vi "PTSequencer.add step.vi"(0 "i ref in":refnum<vi>, 2 "Step":T1, 3 "ms timeout (10000)":i32=10000, 5 "error in (no error)":errorcluster) -> (14 "i ref out":refnum<vi>, 17 "timed out":bool, 19 "error out":errorcluster)   [LabVIEW 2014, in "PTSequencer.lvlib"]
uses:
  PTSequencer.lvlib
  PTSequencer.step.ctl
  CS_Core/CSSystem/CoreDefs/CoreDefs.rawDataType.ctl
  PTSequencer.DIM service condition.ctl
  CS_Core/CSSystem/CoreDefs/CoreDefs.error_type.ctl
  CS_Core/CSSystem/CoreDefs/CoreDefs.error_severity.ctl
  CS_Core/CSSystem/CSSystemLib/CSSystemLib.lvlib
  CS_Core/CSSystem/CoreLib/CoreLib.lvlib
  CS_Core/CSSystem/CoreLib/CoreLib.string 2 byte array.vi
  CS_Core/BaseProcess/BaseProcess.lvlib
  CS_Core/CSSystem/CoreLib/CoreLib.byte array 2 short.vi
  CSlibraries/UtilityLib/UtilityLib.lvlib
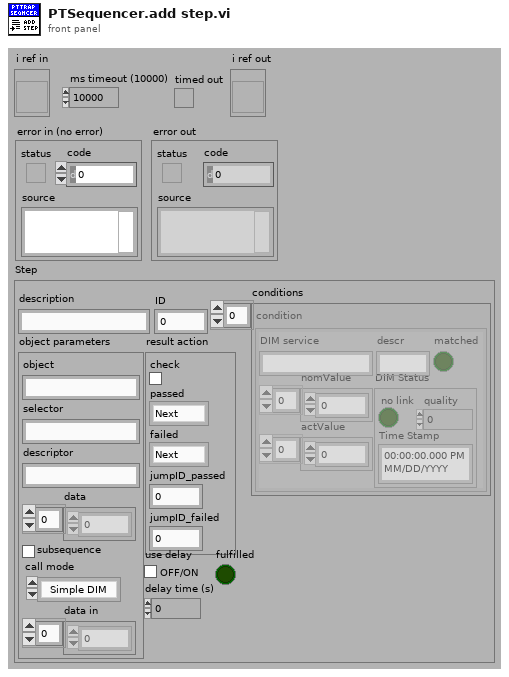
[diagram p1: front panel]
types:
  T1 = typedef "PTSequencer.lvlib/PTSequencer.step.ctl" = cluster{"description":string, "object parameters":cluster{"object":string, "selector":string, "descriptor":string, "data":T2, "subsequence":bool, "call mode":enum16{"Simple DIM", "Synchronous"}, "data in":T2}, "result action":cluster{"check":bool, "passed":enum16{"Next", "Previous", "Repeat", "Jump"}, "failed":enum16{"Next", "Previous", "Repeat", "Jump"}, "jumpID_passed":i32, "jumpID_failed":i32}, "conditions":T3[], "fulfilled ":bool, "use delay":bool, "delay time (s)":dbl, "ID":i32}
  T2 = typedef "CoreDefs.rawDataType.ctl" = i8[]
  T3 = typedef "PTSequencer.lvlib/PTSequencer.DIM service condition.ctl" = cluster{"DIM service":string, "descr":string, "nomValue":T2, "actValue":T2, "matched":bool, "DIM Status":cluster{"no link":bool, "quality":i32, "Time Stamp":timestamp}}
  T4 = typedef "CoreDefs.error_severity.ctl" = enum16{"undefined", "information", "warning", "error", "fatal"}
  T5 = typedef "CoreDefs.error_type.ctl" = enum16{"no error", "can't load process", "can't unload process", "process does not exist", "can't install process", "can't remove process", "unknown function", "time out", "can't execute function", "duplicate queue name", "super not found", "caller queue invalid", "can't ping process", "unknown error", "VISA Error", "VISA timeout", "GPIB timeout", "GPIB error", "communication error", "data type mismatch", "can't read data from OPC server", "can't write data to OPC server", "OET error", "function not implemented", "process already exists", "invalid Shared Variable name", "error writing Shared Variable", "error reading Shared Variable", "invalid client name", "corrupt database", "unknown class", "call not authorized", "parameter out of range", "OET timeout: can't get data to modify", "invalid queue name", "requested operation incompatible with current state", "event undefined", "event disabled", "state undefined", "caller is not a friend", "EventBuilder: bad eventID", "EventBuilder: no DAQ devices", "a thread must not stop itself", "UNUSED ELEMENT4", "DiscArchiver: eventData incomplete", "DiscArchiver: eventData does not belong to run", "DiscArchiver: can't open file", "DiscArchiver: can't write to file", "DiscArchiver: available disc space low", "can't acquire semaphore", "error reading data from database", "notifier object is not existing", "can't register process", "can't unregister process", "illegal event type", "object disabled", "object already exists", "can't change state", "Instrument not found", "no connection to remote node", "invalid reference", "N/A", "UNUSED ELEMENT 1", "element not found", "illegal TCP/IP connection detected", "object does not exist", "invalid access ID", "unknown CS system", "invalid privilige", "unsupported data type", "unsupported server type", "IO server already exists", "Shared Variable already exists"}
  T6 = typedef "PTSequencer.lvlib/PTSequencer.i attribute.ctl" = cluster{"subsequence":bool, "mode":T7, "i step":i32, "nofLoops":i32, "i loop":i32, "Running":bool, "Paused":bool, "step done":bool, "loop done":bool, "seq done":bool, "DIM IDs":cluster{"step done":i32, "loop done":i32, "seq done":i32, "i step":i32, "i loop":i32}, "use stop conditions":bool, "stop conditions":T3[], "Step List":T1[], "DIM subsriptions":string[], "stop cond indexes":i32[], "step cond indexes":cluster{"step condition IDs":cluster{"step ID":i32, "condition ID":i32}[]}[], "Delay Start Time":timestamp, "status":string, "stopping":bool}
  T7 = typedef "PTSequencer.lvlib/PTSequencer.mode.ctl" = enum16{"single", "loop", "for loop"}
  T8 = typedef "CoreDefs.call_type.ctl" = cluster{"Object":string, "Selector":string, "CallType":enum16{"simple", "synchronous", "asynchronous"}, "Async Object":string, "Async Selector":string, "Data Descriptor":T9, "Data":T2, "Error #":i32, "Expire":u32}
  T9 = typedef "BaseProcess.lvlib/BaseProcess.descriptor string definition.ctl" = string
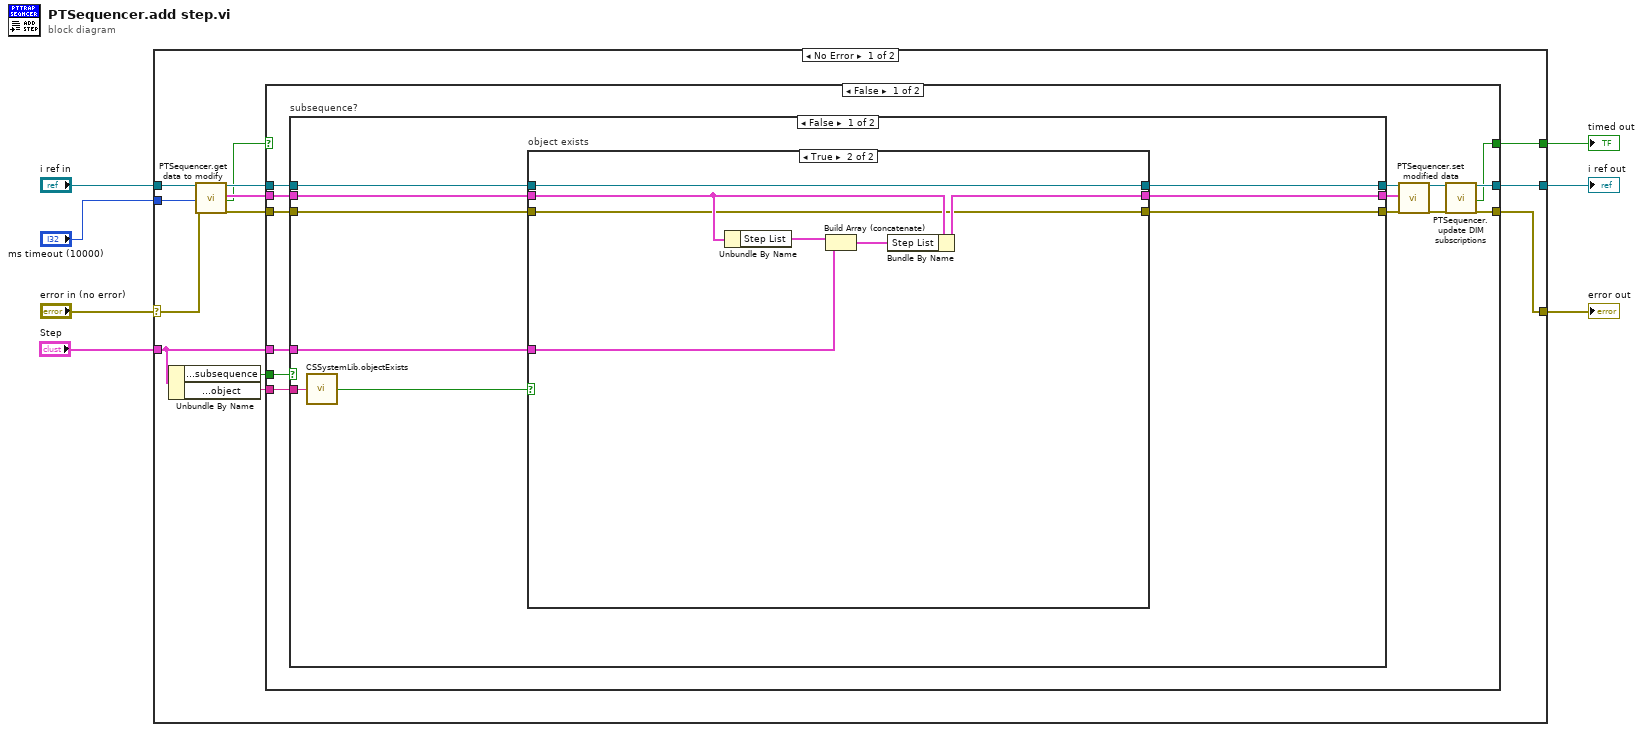
[diagram p0: block diagram]
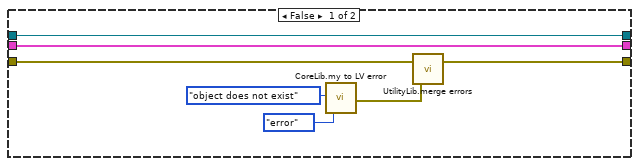
[diagram p2: hidden frame]
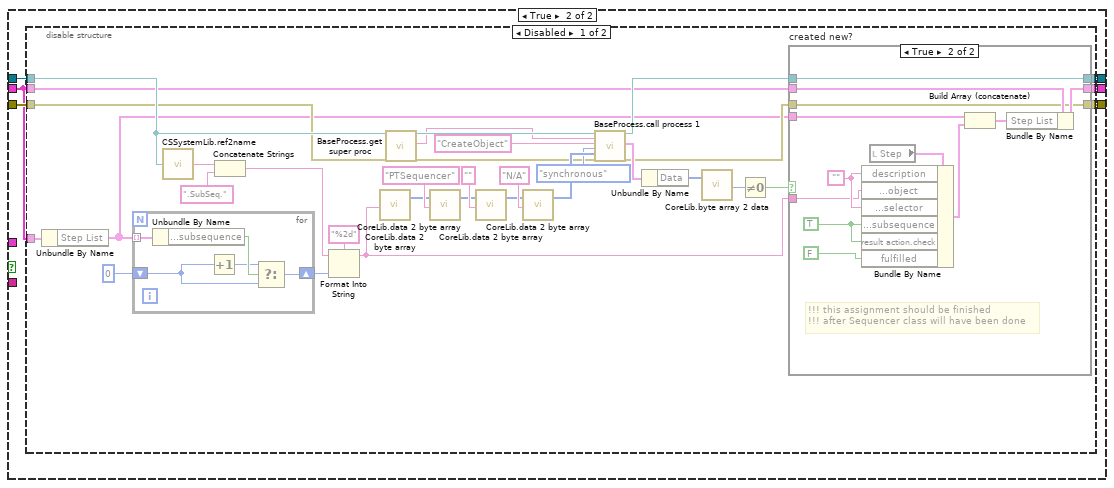
[diagram p3: hidden frame]
diagram:
  n1 = case shown="No Error" "error in (no error)" {
    selector: "error in (no error)" -> [w15 w122]
    tunnel: "i ref in" -> [w20 w123]
    tunnel: [w8 w123] -> w6
    tunnel: "ms timeout (10000)" -> [w11 _]
    tunnel: [w9 w122] -> w3
    tunnel: "Step" -> [w12 _]
    tunnel: [w10 _] -> w1
    frame No Error {
      n2 = Unbundle By Name(w12) -> ("object parameters.subsequence"=w14:bool, "object parameters.object"=w13:string)
      n3 = call "PTSequencer.get data to modify.vi"("i ref in"=w20, "ms timeout (10000)"=w11, "error in (no error)"=w15) -> ("i ref out"=w18:refnum<vi>, "i attribute"=w19:T6, "timed out"=w16:bool, "error out"=w17:errorcluster)  [unwired: 13 in]
      n4 = case shown="False" w16 {
        selector: w16 -> [_ w119]
        tunnel: w19 -> [w34 _]
        tunnel: w18 -> [w33 w121]
        tunnel: w17 -> [w32 w120]
        tunnel: [w23 w121] -> w8
        tunnel: [w22 w120] -> w9
        tunnel: w14 -> [w28 _]
        tunnel: w13 -> [w27 _]
        tunnel: w12 -> [w26 _]
        tunnel: [w21 w119] -> w10
        frame False {
          n5 = case "subsequence?" shown="False" w28 {
            tunnel: w34 -> [w42 w58]
            tunnel: w33 -> [w40 w63]
            tunnel: w32 -> [w38 w60]
            tunnel: [w41 w62] -> w31
            tunnel: [w39 w61] -> w30
            tunnel: [w37 w59] -> w29
            tunnel: w27 -> [w36 _]
            tunnel: w26 -> [w35 _]
            frame False {
              n6 = call "CSSystemLib.objectExists.vi"("name"=w36) -> ("obj exists"=w43:bool)
              n7 = case "object exists" shown="True" w43 {
                tunnel: w42 -> [w50 w56]
                tunnel: [w50 w57] -> w41
                tunnel: w40 -> [w49 w52]
                tunnel: [w49 w52] -> w39
                tunnel: w38 -> [w48 w53]
                tunnel: [w47 w53] -> w37
                tunnel: w35 -> [_ w51]
                frame False {
                  n8 = call "CoreLib.my to LV error.vi"("ErrorTypes"=CoreDefs.error_type."object does not exist", "severityLevel"=CoreDefs.error_severity."error") -> ("myErrorCluster"=w44:errorcluster)  [unwired: 16 in, 1 out]
                  n9 = call "UtilityLib.merge errors.vi"("error2 (no error)"=w44, "error1 (no error)"=w48) -> ("error out"=w47:errorcluster)
                }
                frame True {
                  n10 = Unbundle By Name(w56) -> ("Step List"=w55:T1[])
                  n11 = Build Array (concatenate)(w55, w51) -> (w54:T1[])
                  n12 = Bundle By Name(cluster=w56, "Step List"=w54) -> (w57:T6)
                }
              }
            }
            frame True {
              n13 = disable-structure shown="Disabled" {
                disable-tunnel: w63 -> [w74 w118]
                disable-tunnel: w58 -> [w72 _]
                disable-tunnel: [w71 w116] -> w62
                disable-tunnel: [w70 w118] -> w61
                disable-tunnel: w60 -> [w69 w117]
                disable-tunnel: [w66 w117] -> w59
                disable-tunnel: w58 -> [_ w116]
                frame Disabled {
                  n14 = Unbundle By Name(w72) -> ("Step List"=w65:T1[])
                  n15 = for {
                    tunnel: w65 -> [w115] mode=indexing
                    shift-right: [w111] -> w93
                    shift-left: 0 -> [w112]
                    n16 = Unbundle By Name(w115) -> ("object parameters.subsequence"=w114:bool)
                    n17 = Increment(x=w112) -> (x+1=w113:i32)
                    n18 = Select(t=w113, s=w114, f=w112) -> (s? t:f=w111:i32)
                  }
                  n19 = call "CSSystemLib.ref2name.vi"("obj refnum"=w74) -> ("name"=w92:string)
                  n20 = Concatenate Strings(w92, ".SubSeq.") -> (w90:string)
                  n21 = Format Into String(format string="%2d", initial string=w90, w93) -> (resulting string=w64:string)  [unwired: 1 in, 1 out]
                  n22 = call-poly "CoreLib.data 2 byte array.vi"("string"=w64) -> ("byteArray out"=w83:T2)  [unwired: 18 in]
                  n23 = call "BaseProcess.get super proc.vi"("i ref in"=w74, "error in (no error)"=w69) -> ("i ref out"=w81:refnum<vi>, "SuperProc"=w80:string, "error out"=w68:errorcluster)  [unwired: 15 in]
                  n24 = call-poly "CoreLib.data 2 byte array.vi"("byteArray"=w83, "string"="PTSequencer") -> ("byteArray out"=w84:T2)  [unwired: 17 in]
                  n25 = call-poly "CoreLib.data 2 byte array.vi"("byteArray"=w84, "string"="") -> ("byteArray out"=w85:T2)  [unwired: 17 in]
                  n26 = call-poly "CoreLib.data 2 byte array.vi"("byteArray"=w85, "string"="N/A") -> ("byteArray out"=w87:T2)  [unwired: 17 in]
                  n27 = call "BaseProcess.call process 1.vi"("i ref in"=w81, "Object"=w80, "Selector"="CreateObject", "CallType"=enum16{"simple", "synchronous", "asynchronous"}."synchronous", "Data"=w87, "error in (no error)"=w68) -> ("i ref out"=w73:refnum<vi>, "call cluster out"=w78:T8, "error out"=w67:errorcluster)  [unwired: 11 in]
                  n28 = Unbundle By Name(w78) -> ("Data"=w77:T2)
                  n29 = call-poly "CoreLib.byte array 2 data.vi"("byteArray"=w77) -> ("i16"=w76:i16)  [unwired: 16 in, 2 out]
                  n30 = Not Equal To 0?(x=w76) -> (x != 0?=w75:bool)
                  n31 = case "created new?" shown="True" w75 {
                    tunnel: w73 -> [w98 w108]
                    tunnel: w72 -> [w97 w110]
                    tunnel: [w97 w109] -> w71
                    tunnel: [w98 w108] -> w70
                    tunnel: w67 -> [w96 w103]
                    tunnel: [w96 w103] -> w66
                    tunnel: w65 -> [_ w107]
                    tunnel: w64 -> [_ w99]
                    frame False {
                    }
                    frame True {
                      w100 = TRUE
                      w106 = ""
                      # "!!! this assignment should be finished\n!!! after Sequencer class will have been done"
                      n32 = local read "Step"() -> (w102:T1)
                      n33 = Bundle By Name(cluster=w102, "description"=w106, "object parameters.object"=w99, "object parameters.selector"=w106, "object parameters.subsequence"=w100, "result action.check"=w100, "fulfilled"=FALSE) -> (w101:T1)
                      n34 = Build Array (concatenate)(w107, w101) -> (w104:T1[])
                      n35 = Bundle By Name(cluster=w110, "Step List"=w104) -> (w109:T6)
                    }
                  }
                }
                frame Enabled {
                }
              }
            }
          }
          n36 = call "PTSequencer.set modified data.vi"("i ref in"=w30, "CLASS.i attribute"=w31, "error in (no error)"=w29) -> ("i ref out"=w25:refnum<vi>, "error out"=w24:errorcluster)  [unwired: 15 in]
          n37 = call "PTSequencer.update DIM subscriptions.vi"("i ref in"=w25, "error in"=w24) -> ("i ref out"=w23:refnum<vi>, "timed out"=w21:bool, "error out"=w22:errorcluster)  [unwired: 15 in]
        }
        frame True {
        }
      }
    }
    frame Error {
    }
  }
  "error out" <- w3
  "i ref out" <- w6
  "timed out" <- w1
